vi "Flatten.vi"(8 "error in":errorcluster, 9 "Data":T1) -> (0 "error out":errorcluster, 2 "Buffer":u8[](array[numeric]) format="%.0x")   [LabVIEW 2020, in "Discovery.lvlib"]
uses:
  Discovery.lvlib
  Data.ctl
  lv-protoc/LV-Proto/LV-Proto.lvlib
  Service/Service.lvlib
  ServiceType/Enumeration.ctl
  ServiceType/ServiceType.lvlib
  Service/Data.ctl
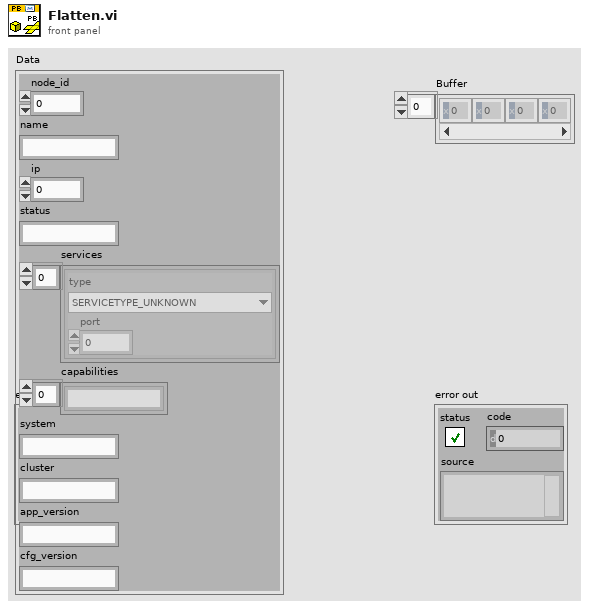
[diagram p1: front panel]
types:
  T1 = typedef "Discovery.lvlib/Data.ctl" = cluster{"node_id":u32, "name":string, "ip":u32, "status":string, "services":T2[], "capabilities":string[], "system":string, "cluster":string, "app_version":string, "cfg_version":string}
  T2 = typedef "Service.lvlib/Data.ctl" = cluster{"type":T3, "port":i32}
  T3 = typedef "ServiceType.lvlib/Enumeration.ctl" = enum16{"SERVICETYPE_UNKNOWN", "SERVICETYPE_TCPSERVER", "SERVICETYPE_HTTPSERVER"}
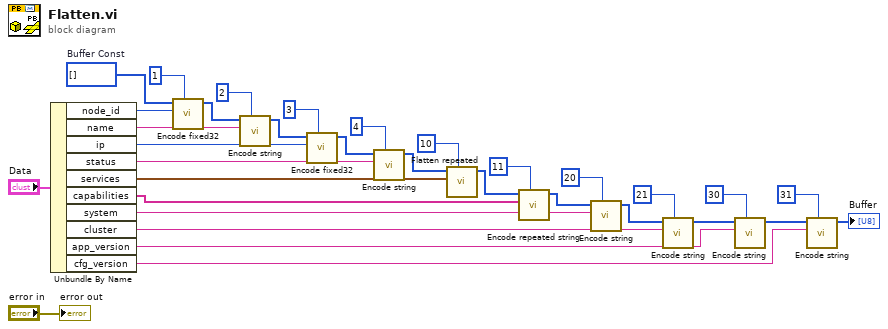
[diagram p0: block diagram]
diagram:
  w31 = u8[] []  # Buffer Const
  n1 = Unbundle By Name("Data") -> ("node_id"=w29:u32, "name"=w26:string, "ip"=w23:u32, "status"=w20:string, "services"=w18:T2[], "capabilities"=w14:string[], "system"=w11:string, "cluster"=w8:string, "app_version"=w5:string, "cfg_version"=w2:string)
  n2 = call "Encode fixed32.vi"("Field Number"=1, "fixed32"=w29, "Buffer in"=w31) -> ("Buffer"=w28:u8[])  [unwired: 8 in]
  n3 = call "Encode string.vi"("Field Number"=2, "string"=w26, "Buffer in"=w28) -> ("Buffer"=w25:u8[])  [unwired: 8 in]
  n4 = call "Encode fixed32.vi"("Field Number"=3, "fixed32"=w23, "Buffer in"=w25) -> ("Buffer"=w22:u8[])  [unwired: 8 in]
  n5 = call "Encode string.vi"("Field Number"=4, "string"=w20, "Buffer in"=w22) -> ("Buffer"=w19:u8[])  [unwired: 8 in]
  n6 = call "Flatten repeated.vi"("Field Number"=10, "Data"=w18, "Buffer in"=w19) -> ("Buffer"=w16:u8[])  [unwired: 8 in]
  n7 = call "Encode repeated string.vi"("Field Number"=11, "string"=w14, "Buffer in"=w16) -> ("Buffer"=w13:u8[])  [unwired: 8 in]
  n8 = call "Encode string.vi"("Field Number"=20, "string"=w11, "Buffer in"=w13) -> ("Buffer"=w10:u8[])  [unwired: 8 in]
  n9 = call "Encode string.vi"("Field Number"=21, "string"=w8, "Buffer in"=w10) -> ("Buffer"=w7:u8[])  [unwired: 8 in]
  n10 = call "Encode string.vi"("Field Number"=30, "string"=w5, "Buffer in"=w7) -> ("Buffer"=w4:u8[])  [unwired: 8 in]
  n11 = call "Encode string.vi"("Field Number"=31, "string"=w2, "Buffer in"=w4) -> ("Buffer"=→"Buffer":u8[])  [unwired: 8 in]
  "error out" <- "error in"
